vi "get_path_group.vi"(8 "error in (no error)":errorcluster, 11 "Experiments_group.lvclass in":refnum<class "Experiments_group.lvclass">) -> (0 "error out":errorcluster, 2 "Path":path, 3 "Experiments_group.lvclass out":refnum<class "Experiments_group.lvclass">)   [LabVIEW 2015, in "Experiments_group.lvclass"]
uses:
  Experiments_group.lvclass
  Experiments_group.lvclass/Experiments_group.ctl
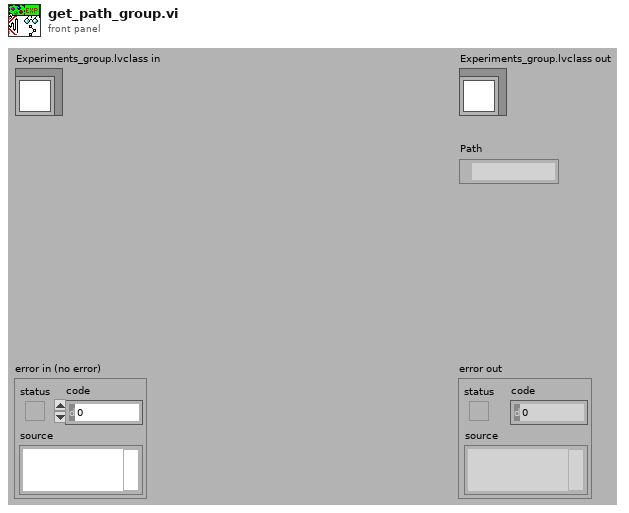
[diagram p1: front panel]
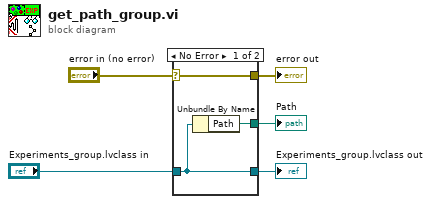
[diagram p0: block diagram]
diagram:
  n1 = case shown="No Error" "error in (no error)" {
    selector: "error in (no error)" -> [w8 w9]
    tunnel: [w8 w9] -> w4
    tunnel: [w7 w10] -> w2
    tunnel: "Experiments_group.lvclass in" -> [w7 w10]
    tunnel: [w6 _] -> w1
    frame No Error {
      n2 = Unbundle By Name(w7) -> ("Path"=w6:path)
    }
    frame Error {
    }
  }
  "error out" <- w4
  "Experiments_group.lvclass out" <- w2
  "Path" <- w1
